vi "CirclePosition.vi"() -> ()   [LabVIEW 2016]
uses:
  <vilib>/userdefined/High Color/IMAQdx.ctl
  <vilib>/vision/driver/NI_Vision_Acquisition_Software.lvlib
panel:
  in  "stop":bool
  out "Circle Descriptor":T1(array[cluster])
  out "Image":T2(plugin-control)
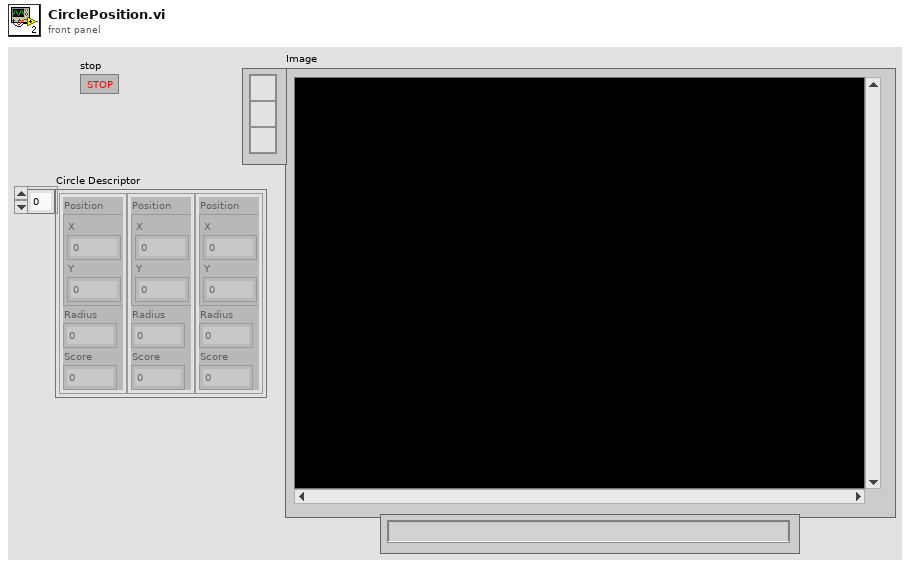
[diagram p1: front panel]
types:
  T1 = cluster{"Position":cluster{"X":sgl, "Y":sgl}, "Radius":dbl, "Score":dbl}[]
  T2 = typedef "IMAQ Image.ctl" = refnum<image>
  T3 = typedef "IMAQdx.ctl" = refnum<k21>
  T4 = typedef "Image Type" = u32
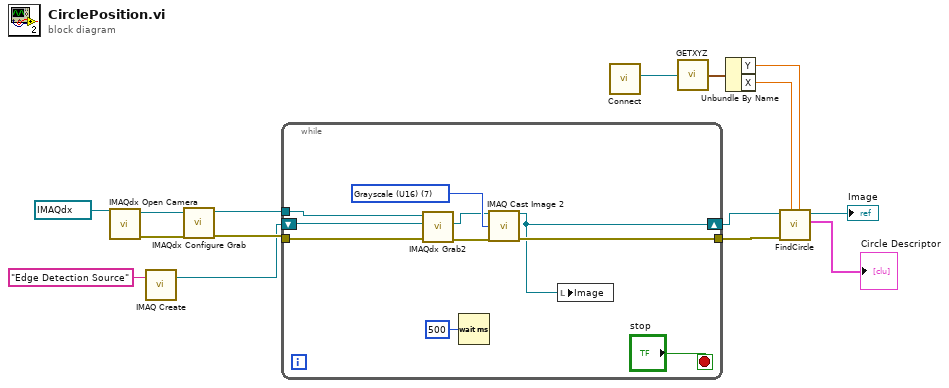
[diagram p0: block diagram]
diagram:
  n1 = call <vilib>:"IMAQdx Open Camera.vi"("Session In"=T3 "cam0") -> ("error out"=w9:errorcluster, "Session Out"=w10:T3)  [unwired: 9 in]
  n2 = call "IMAQ Create"("Image Name"="Edge Detection Source") -> ("New Image"=w2:T2)  [unwired: 4 in, 1 out]
  n3 = call <vilib>:"IMAQdx Configure Grab.vi"("error in"=w9, "Session In"=w10) -> ("error out"=w8:errorcluster, "Session Out"=w3:T3)  [unwired: 8 in]
  n4 = while {
    tunnel: w8 -> [w25]
    tunnel: [w23] -> w7
    tunnel: w3 -> [w20]
    shift-right: [w18] -> w1
    shift-left: w2 -> [w19]
    stop <- "stop" stop-if-true
    w22 = T4 7 items=["Grayscale (U8)", "Grayscale (I16)", "Grayscale (SGL)", "Complex (CSG)", "RGB (U32)", "HSL (U32)", "RGB (U64)", "Grayscale (U16)"] ("Image Type")
    n5 = call <vilib>:"IMAQdx Grab2.vi"("error in"=w25, "Image In"=w19, "Session In"=w20) -> ("error out"=w24:errorcluster, "Image Out"=w21:T2)  [unwired: 5 in, 2 out]
    n6 = Wait (ms)(milliseconds to wait=u32 500) -> ()  [unwired: 1 out]
    n7 = call "IMAQ Cast Image 2"("Image Src"=w21, "Image Type"=w22, "error in (no error)"=w24) -> ("Image Dst Out"=w18:T2, "error out"=w23:errorcluster)  [unwired: 11 in]
    n8 = local write "Image"(w18) -> ()
  }
  n9 = call "Connect.vi"() -> ("controller"=w15:refnum<k24>)  [unwired: 10 in, 1 out]
  n10 = call "GETXYZ.vi"(".NET Refnum in"=w15) -> ("XYZ"=w14:cluster{"X":dbl, "Y":dbl, "Z":dbl})
  n11 = Unbundle By Name(w14) -> ("Y"=w13:dbl, "X"=w12:dbl)
  n12 = call "FindCircle.vi"("Y"=w13, "X"=w12, "error in (no error)"=w7, "Image 2"=w1) -> ("Circle Descriptor"=→"Circle Descriptor":T1, "Image Out"=→"Image":T2)  [unwired: 5 in, 1 out]
